vi "Teleop.vi"(10 "Match Info":T1={"Autonomous Elapsed Seconds"=0.0, "TeleOp Elapsed Seconds"=0.0, "Disabled Elapsed Seconds"=0.0, "Visited Autonomous"=FALSE, "Visited TeleOp"=FALSE, "Visited Disabled"=FALSE, "Autonomous Settings"={"Autonomous Style"=enum."Independent", "VI Refnum"=refnum}}, 11 "Call Context":T2) -> ()   [LabVIEW 2017]
doc: "This VI is called for each TeleOp packet received from the DS where the robot is not disabled. It is often used to read from the joysticks and update I/O or to update setpoints for timed control loops. It should complete and return within 20 milliseconds or it may miss DS packets."
uses:
  <vilib>/Rock Robotics/WPI/DriverStation/WPI_DriverStationDerivedRobotMode.ctl
  <vilib>/Rock Robotics/WPI/DriverStation/WPI_DriverStationMatch Info.ctl
  <vilib>/Rock Robotics/WPI/Solenoid/WPI_SolenoidValue.ctl
  <vilib>/Rock Robotics/WPI/Utilities/WPI_GetSetVariantRefNum.vi
  <vilib>/Rock Robotics/Network Tables/NT Write Boolean Array.vi
  <vilib>/Rock Robotics/Network Tables/NT Write Numeric Array.vi
  <vilib>/Rock Robotics/Network Tables/NT Read Boolean.vi
  <vilib>/Rock Robotics/Network Tables/NT Read Number.vi
  Robot Global Data.vi
  <vilib>/Rock Robotics/WPI/ThirdParty/Phoenix-LabVIEW/Motor Controller/Get/CTRE_Phoenix_MotorController_GetQuadratureData.vi
  <vilib>/Rock Robotics/WPI/Solenoid/WPI_SolenoidSetEnum.vi
  <vilib>/Rock Robotics/WPI/RobotDrive/WPI_RobotDriveArcadeDrive_Standard(NoSaturation).vi
panel:
  out "Quadrature Velocity":i32
  out "height":dbl
  out "Quadrature Position":i32
  out "Sample Slider 0":dbl(slide) scale=0.0..5.0
  out "Sample Boolean 1":bool
  out "Sample Boolean 0":bool
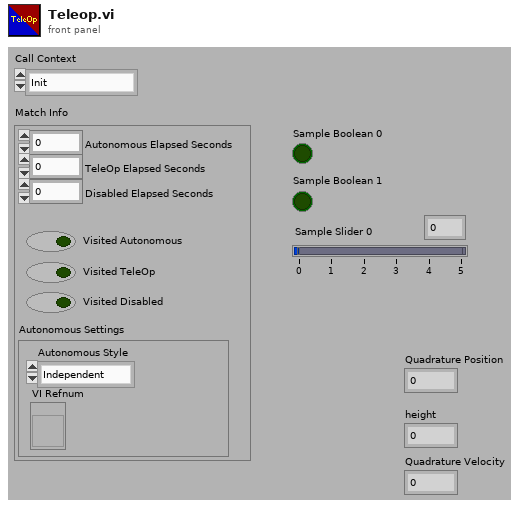
[diagram p1: front panel]
types:
  T1 = typedef "WPI_DriverStationMatch Info.ctl" = cluster{"Autonomous Elapsed Seconds":dbl, "TeleOp Elapsed Seconds":dbl, "Disabled Elapsed Seconds":dbl, "Visited Autonomous":bool, "Visited TeleOp":bool, "Visited Disabled":bool, "Autonomous Settings":cluster{"Autonomous Style":enum16{"Iterative", "Independent"}, "VI Refnum":refnum<vi>}}
  T2 = typedef "WPI_DriverStationDerivedRobotMode.ctl" = enum16{"Init", "Execute", "Stop"}
  T3 = typedef "WPI_SolenoidValue.ctl" = enum16{"Off", "On", "Forward", "Reverse"}
  T4 = typedef "WPI_JoystickDevRef.ctl" = cluster{"Device":T5}
  T5 = typedef "WPI_JoystickDeviceEnum.ctl" = enum16{"USB 0", "USB 1", "USB 2", "USB 3", "USB 4", "USB 5"}
  T6 = typedef "WPI_RobotDriveDevRef.ctl" = cluster{"DevStatus":errorcluster, "Motors[]":T7[], "Square Inputs":bool, "Max Output":dbl}
  T7 = typedef "WPI_MotorControlDeviceRef.ctl" = cluster{"DeviceStatus":errorcluster, "Type":T8, "PWM":cluster{"PWM Channel":T9, "DeadBand":T10}, "CAN":cluster{"Device Number":u8, "SetOutput VI Ref":variant, "GetOutput VI Ref":variant, "Enable VI Ref":variant, "Disable VI Ref":variant, "Data":variant}, "Invert":bool, "DIO PWM":cluster{"PWM \"Enable\" Channel":T9, "DIOChannel":T11, "PWM Rate":dbl}}
  T8 = typedef "WPI_MotorControlType.ctl" = enum16{"PWM", "CAN", "DIO PWM"}
  T9 = typedef "FPGA_DIOPWMChannel.ctl" = enum8{"PWM 0", "PWM 1", "PWM 2", "PWM 3", "PWM 4", "PWM 5", "PWM 6", "PWM 7", "PWM 8", "PWM 9", "PWM MXP 0", "PWM MXP 1", "PWM MXP 2", "PWM MXP 3", "PWM MXP 4", "PWM MXP 5", "PWM MXP 6", "PWM MXP 7", "PWM MXP 8", "PWM MXP 9", "Invalid"}
  T10 = typedef "WPI_PWMDeadband.ctl" = cluster{"Name":string, "maxPositivePwm":i32, "minPositivePwm":i32, "centerPwm":i32, "maxNegativePwm":i32, "minNegativePwm":i32, "angularRange":u16}
  T11 = typedef "FPGA_DIOChannel.ctl" = enum8{"DIO 0", "DIO 1", "DIO 2", "DIO 3", "DIO 4", "DIO 5", "DIO 6", "DIO 7", "DIO 8", "DIO 9", "DIO MXP 0", "DIO MXP 1", "DIO MXP 2", "DIO MXP 3", "DIO MXP 4", "DIO MXP 5", "DIO MXP 6", "DIO MXP 7", "DIO MXP 8", "DIO MXP 9", "DIO MXP 10", "DIO MXP 11", "DIO MXP 12", "DIO MXP 13", "DIO MXP 14", "DIO MXP 15", "SPI Port CS1", "SPI Port CS2", "SPI Port CS3", "SPI Port MISO", "SPI Port MOSI", "Invalid"}
  T12 = cluster{"Yaw":dbl, "Roll":dbl, "Pitch":dbl, "Heading":dbl, "Fused Heading":dbl}
  T13 = typedef "WPI_SolenoidDevRef.ctl" = cluster{"DevStatus":errorcluster, "Pneumatics Control Module":u8, "Forward Solenoid Channel":T14, "Reverse Solenoid Channel":T14}
  T14 = typedef "WPI_SolenoidChannel.ctl" = enum8{"Solenoid 0", "Solenoid 1", "Solenoid 2", "Solenoid 3", "Solenoid 4", "Solenoid 5", "Solenoid 6", "Solenoid 7", "Invalid"}
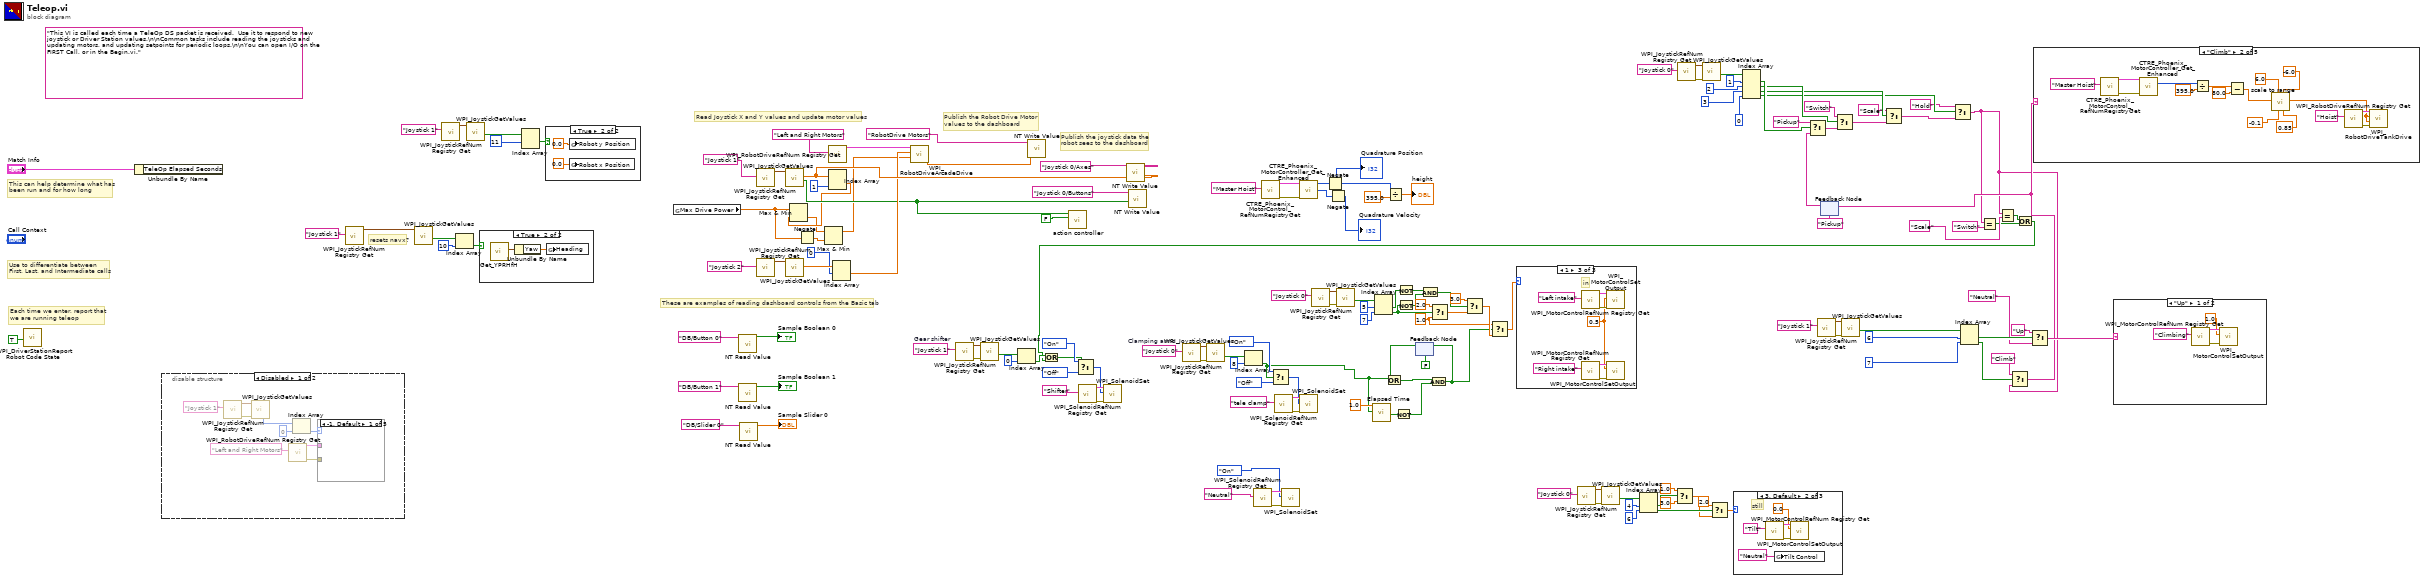
[diagram p0: block diagram]
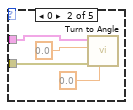
[diagram p2: hidden frame]
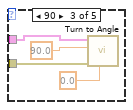
[diagram p3: hidden frame]
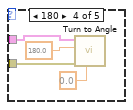
[diagram p4: hidden frame]
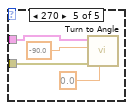
[diagram p5: hidden frame]
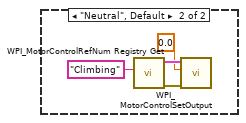
[diagram p7: hidden frame]
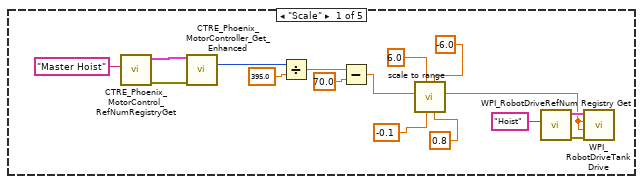
[diagram p8: hidden frame]
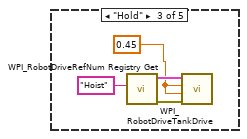
[diagram p9: hidden frame]
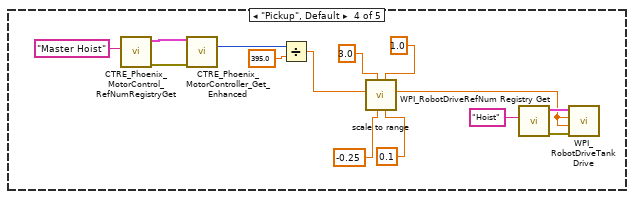
[diagram p10: hidden frame]
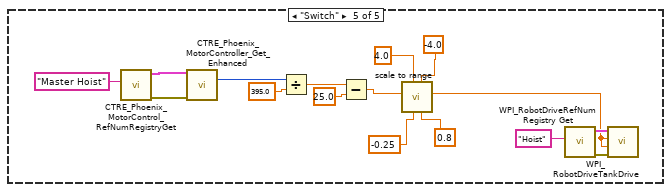
[diagram p11: hidden frame]
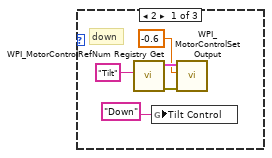
[diagram p12: hidden frame]
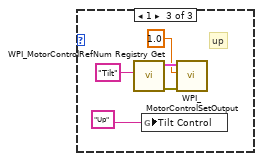
[diagram p13: hidden frame]
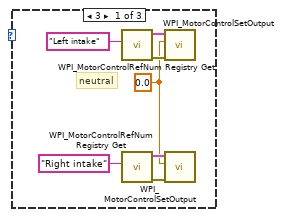
[diagram p14: hidden frame]
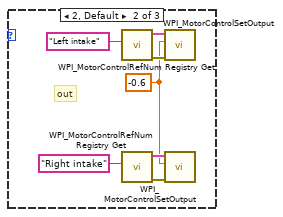
[diagram p15: hidden frame]
diagram:
  w74 = "Joystick 0"  # Clamping arms
  w65 = 1.0 ("f")
  w122 = "Joystick 1"  # Gear shifter
  (unwired) "This VI is called each time a TeleOp DS packet is received.  Use it to respond to new joystick or Driver Station values.\n\nCommon tasks include reading the joysticks and updating motors, and updating setpoints for periodic loops.\n\nYou can open I/O on the FIRST Call, or in the Begin.vi."
  # "resets navx?"
  # "These are examples of reading dashboard controls from the Basic tab"
  # "Publish the Robot Drive Motor\nvalues to the dashboard"
  # "Publish the joystick data the\nrobot sees to the dashboard"
  # "Each time we enter, report that\nwe are running teleop"
  # "Use to differentiate between\nFirst, Last, and Intermediate calls"
  # "This can help determine what has\nbeen run and for how long"
  # "Read Joystick X and Y values and update motor values"
  n1 = call <vilib>:"WPI_DriverStationReport Robot Code State.vi"("TeleOp"=TRUE ("Autonomous")) -> ()  [unwired: 10 in, 1 out]
  n2 = Unbundle By Name("Match Info") -> ()  [unwired: 1 out]
  n3 = disable-structure shown="Disabled" {
    frame Disabled {
      n4 = call <vilib>:"WPI_JoystickRefNum Registry Get.vi"("refnum name"="Joystick 1") -> ("error out"=w156:errorcluster, "JoystickDevRef"=w163:T4)  [unwired: 1 in, 8 out]
      n5 = call <vilib>:"WPI_JoystickGetValues.vi"("error in (no error)"=w156, "JoystickDevRef"=w163) -> ("POVs"=w157:i16[])  [unwired: 5 in, 4 out]
      n6 = call <vilib>:"WPI_RobotDriveRefNum Registry Get.vi"("refnum name"="Left and Right Motors") -> ("error out"=w160:errorcluster, "RobotDriveDevRef"=w159:T6)  [unwired: 1 in, 8 out]
      n7 = Index Array(array=w157, index=0) -> (element=w158:i16)
      n8 = case shown="-1, Default" w158 {
        tunnel: w160 -> [_ w166 w169 w175 w178]
        tunnel: w159 -> [_ w165 w170 w174 w177]
        frame -1, Default {
        }
        frame 0 {
          n9 = call "Turn to Angle.vi"("in power"=0.0, "error in (no error)"=w166, "Angle"=0.0, "RobotDriveDevRef"=w165) -> ()  [unwired: 5 in, 3 out]
        }
        frame 90 {
          n10 = call "Turn to Angle.vi"("in power"=0.0, "error in (no error)"=w169, "Angle"=90.0, "RobotDriveDevRef"=w170) -> ()  [unwired: 5 in, 3 out]
        }
        frame 180 {
          n11 = call "Turn to Angle.vi"("in power"=0.0, "error in (no error)"=w175, "Angle"=180.0, "RobotDriveDevRef"=w174) -> ()  [unwired: 5 in, 3 out]
        }
        frame 270 {
          n12 = call "Turn to Angle.vi"("in power"=0.0, "error in (no error)"=w178, "Angle"=-90.0, "RobotDriveDevRef"=w177) -> ()  [unwired: 5 in, 3 out]
        }
      }
    }
    frame Enabled {
    }
  }
  n13 = call <vilib>:"WPI_JoystickRefNum Registry Get.vi"("refnum name"="Joystick 1") -> ("JoystickDevRef"=w132:T4)  [unwired: 1 in, 9 out]
  n14 = call <vilib>:"WPI_JoystickGetValues.vi"("JoystickDevRef"=w132) -> ("Buttons"=w130:bool[])  [unwired: 6 in, 4 out]
  n15 = call <vilib>:"WPI_JoystickRefNum Registry Get.vi"("refnum name"="Joystick 1") -> ("JoystickDevRef"=w126:T4)  [unwired: 1 in, 9 out]
  n16 = Index Array(array=w130, index=10) -> (element=w129:bool)
  n17 = call <vilib>:"WPI_JoystickGetValues.vi"("JoystickDevRef"=w126) -> ("Buttons"=w124:bool[])  [unwired: 6 in, 4 out]
  n18 = case shown="True" w129 {
    frame False {
    }
    frame True {
      n19 = call <vilib>:"Get_YPRHfH.vi"() -> ("YRPHfH"=w182:T12)  [unwired: 11 in]
      n20 = Unbundle By Name(w182) -> ("Yaw"=w181:dbl)
      n21 = global write "Robot Global Data.vi" "Heading"(w181) -> ()
    }
  }
  n22 = Index Array(array=w124, index #1=11 ("index")) -> (element #1=w123:bool)  [unwired: 1 in, 1 out]
  n23 = case shown="True" w123 {
    frame False {
    }
    frame True {
      n24 = global write "Robot Global Data.vi" "Robot y Position"(0.0 ("Robot y Position")) -> ()
      n25 = global write "Robot Global Data.vi" "Robot x Position"(0.0 ("Robot x Position")) -> ()
    }
  }
  n26 = global read "Robot Global Data.vi" "Max Drive Power"() -> (w29:dbl)
  n27 = call-poly <vilib>:"NT Read Value.vi"("Name"="DB/Button 0" ("refnum name")) -> ("Boolean"=→"Sample Boolean 0":bool)  [unwired: 9 in, 1 out]
  n28 = call-poly <vilib>:"NT Read Value.vi"("Name"="DB/Button 1" ("refnum name")) -> ("Boolean"=→"Sample Boolean 1":bool)  [unwired: 9 in, 1 out]
  n29 = call-poly <vilib>:"NT Read Value.vi"("Name"="DB/Slider 0" ("refnum name")) -> ("Numeric"=→"Sample Slider 0":dbl)  [unwired: 9 in, 1 out]
  n30 = call <vilib>:"WPI_JoystickRefNum Registry Get.vi"("refnum name"="Joystick 1") -> ("JoystickDevRef"=w151:T4)  [unwired: 1 in, 9 out]
  n31 = call <vilib>:"WPI_JoystickRefNum Registry Get.vi"("refnum name"="Joystick 2") -> ("JoystickDevRef"=w136:T4)  [unwired: 1 in, 9 out]
  n32 = call <vilib>:"WPI_JoystickGetValues.vi"("JoystickDevRef"=w151) -> ("Buttons"=w78:bool[], "Axes"=w147:dbl[])  [unwired: 6 in, 3 out]
  n33 = call <vilib>:"WPI_JoystickGetValues.vi"("JoystickDevRef"=w136) -> ("Axes"=w135:dbl[])  [unwired: 6 in, 4 out]
  n34 = Negate(x=w29) -> (-x=w30:dbl)
  n35 = call <vilib>:"WPI_RobotDriveRefNum Registry Get.vi"("refnum name"="Left and Right Motors") -> ("RobotDriveDevRef"=w153:T6)  [unwired: 1 in, 9 out]
  n36 = Index Array(array=w147, index #1=1 ("index")) -> (element #1=w28:dbl)  [unwired: 1 in, 1 out]
  n37 = Max & Min(x=w29, y=w28) -> (min(x,y)=w27:dbl)  [unwired: 1 out]
  n38 = Max & Min(x=w27, y=w30) -> (max(x,y)=w26:dbl)  [unwired: 1 out]
  n39 = Index Array(array=w135, index #1=0 ("index")) -> (element #1=w112:dbl)  [unwired: 1 in, 1 out]
  n40 = call-poly <vilib>:"WPI_RobotDriveArcadeDrive.vi"("Y axis value"=w26, "X axis value"=w112, "RobotDriveDevRef"=w153) -> ("Motor Values"=w141:dbl[])  [unwired: 6 in, 2 out]
  n41 = call <vilib>:"WPI_JoystickRefNum Registry Get.vi"("refnum name"=w122) -> ("error out"=w81:errorcluster, "JoystickDevRef"=w121:T4)  [unwired: 1 in, 8 out]
  n42 = call <vilib>:"WPI_JoystickGetValues.vi"("error in (no error)"=w81, "JoystickDevRef"=w121) -> ("Buttons"=w119:bool[])  [unwired: 5 in, 4 out]
  n43 = Index Array(array=w119, index=0) -> (element=w15:bool)
  n44 = call-poly <vilib>:"NT Write Value.vi"("Numeric Array"=w141, "Name"="RobotDrive Motors") -> ()  [unwired: 9 in, 1 out]
  n45 = call "action controller.vi"("Box Sensor"=FALSE, "Buttons"=w78) -> ()  [unwired: 10 in]
  n46 = call <vilib>:"WPI_SolenoidRefNum Registry Get.vi"("refnum name"="Shifter") -> ("error out"=w118:errorcluster, "SolenoidDevRef"=w117:T13)  [unwired: 9 in]
  n47 = call-poly <vilib>:"NT Write Value.vi"("Numeric Array"=w147, "Name"="Joystick 0/Axes") -> ()  [unwired: 9 in, 1 out]
  n48 = call-poly <vilib>:"NT Write Value.vi"("Boolean Array"=w78, "Name"="Joystick 0/Buttons") -> ()  [unwired: 9 in, 1 out]
  n49 = call <vilib>:"WPI_JoystickRefNum Registry Get.vi"("refnum name"=w74) -> ("error out"=w72:errorcluster, "JoystickDevRef"=w73:T4)  [unwired: 1 in, 8 out]
  n50 = call <vilib>:"WPI_JoystickGetValues.vi"("error in (no error)"=w72, "JoystickDevRef"=w73) -> ("Buttons"=w71:bool[])  [unwired: 5 in, 4 out]
  n51 = Index Array(array=w71, index=8) -> (element=w1:bool)
  n52 = call <vilib>:"WPI_SolenoidRefNum Registry Get.vi"("refnum name"="Neutral") -> ("error out"=w6:errorcluster, "SolenoidDevRef"=w4:T13)  [unwired: 9 in]
  n53 = call <vilib>:"CTRE_Phoenix_MotorControl_RefNumRegistryGet.vi"("refnum name"="Master Hoist") -> ("error out"=w91:errorcluster, "PhoenixMotorControlDevRef"=w90:T7)  [unwired: 9 in]
  n54 = Select(t=WPI_SolenoidValue."On" ("Value"), s=w1, f=WPI_SolenoidValue."Off" ("Value")) -> (s? t:f=w67:T3)
  n55 = call <vilib>:"WPI_SolenoidRefNum Registry Get.vi"("refnum name"="tele clamp") -> ("error out"=w76:errorcluster, "SolenoidDevRef"=w77:T13)  [unwired: 9 in]
  n56 = call-poly <vilib>:"WPI_SolenoidSet.vi"("error in (no error)"=w6, "Value"=WPI_SolenoidValue."On", "SolenoidDevRef"=w4) -> ()  [unwired: 7 in, 2 out]
  n57 = call-poly <vilib>:"WPI_SolenoidSet.vi"("error in (no error)"=w76, "Value"=w67, "SolenoidDevRef"=w77) -> ()  [unwired: 7 in, 2 out]
  n58 = call-poly <vilib>:"CTRE_Phoenix_MotorController_Get_Enhanced.vi"("PhoenixMotorControlDevRef"=w90, "error in"=w91) -> ("Quadrature Position"=w87:i32, "Quadrature Velocity"=w62:i32)  [unwired: 10 in, 2 out]
  n59 = call <vilib>:"WPI_JoystickRefNum Registry Get.vi"("refnum name"="Joystick 0") -> ("error out"=w93:errorcluster, "JoystickDevRef"=w104:T4)  [unwired: 1 in, 8 out]
  n60 = Negate(x=w87) -> (-x=w40:i32)
  "Quadrature Position" <- w40
  n61 = Negate(x=w62) -> (-x=→"Quadrature Velocity":i32)
  n62 = call <vilib>:"WPI_JoystickGetValues.vi"("error in (no error)"=w93, "JoystickDevRef"=w104) -> ("Buttons"=w103:bool[])  [unwired: 5 in, 4 out]
  n63 = call "Elapsed Time"("Time Target (s)"=1.0, "Reset"=w1) -> ("Time has Elapsed"=w12:bool)  [unwired: 10 in, 7 out]
  n64 = Index Array(array=w103, index #1=5 ("index"), index #2=7 ("index")) -> (element #1=w101:bool, element #2=w95:bool)
  n65 = Divide(x=w40, y=395.0) -> (x/y=→"height":dbl)
  n66 = Not(x=w12) -> (.not. x?=w8:bool)
  n67 = Not(x=w101) -> (.not. x?=w100:bool)
  n68 = Not(x=w95) -> (.not. x?=w98:bool)
  n69 = feedback #1(FALSE) -> (w10:bool)
  n70 = Or(x=w1, y=w10) -> (x .or. y?=w9:bool)
  n71 = And(x=w100, y=w98) -> (x .and. y?=w99:bool)
  n72 = And(x=w9, y=w8) -> (x .and. y?=w7:bool)
  n73 = feedback-in #1(w7) -> ()
  n74 = Select(t=2.0, s=w95, f=w65) -> (s? t:f=w96:dbl)
  n75 = Select(t=3.0, s=w99, f=w96) -> (s? t:f=w66:dbl)
  n76 = Select(t=w65, s=w7, f=w66) -> (s? t:f=w64:dbl)
  n77 = case shown="1" w64 {
    frame 3 {
      w185 = 0.0
      # "neutral"
      n78 = call <vilib>:"WPI_MotorControlRefNum Registry Get.vi"("refnum name"="Left intake") -> ("error out"=w190:errorcluster, "MotorControlDevRef"=w189:T7)  [unwired: 9 in]
      n79 = call <vilib>:"WPI_MotorControlRefNum Registry Get.vi"("refnum name"="Right intake") -> ("error out"=w188:errorcluster, "MotorControlDevRef"=w187:T7)  [unwired: 9 in]
      n80 = call <vilib>:"WPI_MotorControlSetOutput.vi"("error in (no error)"=w190, "Output"=w185, "MotorControlDevRef"=w189) -> ()  [unwired: 6 in, 3 out]
      n81 = call <vilib>:"WPI_MotorControlSetOutput.vi"("error in (no error)"=w188, "Output"=w185, "MotorControlDevRef"=w187) -> ()  [unwired: 6 in, 3 out]
    }
    frame 2, Default {
      w192 = -0.6
      # "out"
      n82 = call <vilib>:"WPI_MotorControlRefNum Registry Get.vi"("refnum name"="Left intake") -> ("error out"=w197:errorcluster, "MotorControlDevRef"=w196:T7)  [unwired: 9 in]
      n83 = call <vilib>:"WPI_MotorControlRefNum Registry Get.vi"("refnum name"="Right intake") -> ("error out"=w195:errorcluster, "MotorControlDevRef"=w194:T7)  [unwired: 9 in]
      n84 = call <vilib>:"WPI_MotorControlSetOutput.vi"("error in (no error)"=w197, "Output"=w192, "MotorControlDevRef"=w196) -> ()  [unwired: 6 in, 3 out]
      n85 = call <vilib>:"WPI_MotorControlSetOutput.vi"("error in (no error)"=w195, "Output"=w192, "MotorControlDevRef"=w194) -> ()  [unwired: 6 in, 3 out]
    }
    frame 1 {
      w199 = 0.5 ("Output")
      # "in"
      n86 = call <vilib>:"WPI_MotorControlRefNum Registry Get.vi"("refnum name"="Left intake") -> ("error out"=w204:errorcluster, "MotorControlDevRef"=w203:T7)  [unwired: 9 in]
      n87 = call <vilib>:"WPI_MotorControlRefNum Registry Get.vi"("refnum name"="Right intake") -> ("error out"=w202:errorcluster, "MotorControlDevRef"=w201:T7)  [unwired: 9 in]
      n88 = call <vilib>:"WPI_MotorControlSetOutput.vi"("error in (no error)"=w204, "Output"=w199, "MotorControlDevRef"=w203) -> ()  [unwired: 6 in, 3 out]
      n89 = call <vilib>:"WPI_MotorControlSetOutput.vi"("error in (no error)"=w202, "Output"=w199, "MotorControlDevRef"=w201) -> ()  [unwired: 6 in, 3 out]
    }
  }
  n90 = call <vilib>:"WPI_JoystickRefNum Registry Get.vi"("refnum name"="Joystick 0") -> ("error out"=w106:errorcluster, "JoystickDevRef"=w110:T4)  [unwired: 1 in, 8 out]
  n91 = call <vilib>:"WPI_JoystickGetValues.vi"("error in (no error)"=w106, "JoystickDevRef"=w110) -> ("Buttons"=w109:bool[])  [unwired: 5 in, 4 out]
  n92 = Index Array(array=w109, index #1=4 ("index"), index #2=6 ("index")) -> (element #1=w86:bool, element #2=w85:bool)
  n93 = Select(t=1.0, s=w86, f=3.0) -> (s? t:f=w80:dbl)
  n94 = call <vilib>:"WPI_JoystickRefNum Registry Get.vi"("refnum name"="Joystick 0") -> ("error out"=w61:errorcluster, "JoystickDevRef"=w60:T4)  [unwired: 9 in]
  n95 = call <vilib>:"WPI_JoystickGetValues.vi"("error in (no error)"=w61, "JoystickDevRef"=w60) -> ("Buttons"=w57:bool[])  [unwired: 5 in, 4 out]
  n96 = Select(t=2.0 ("f"), s=w85, f=w80) -> (s? t:f=w82:dbl)
  n97 = case shown="3, Default" w82 {
    frame 2 {
      # "down"
      n98 = call <vilib>:"WPI_MotorControlRefNum Registry Get.vi"("refnum name"="Tilt") -> ("error out"=w209:errorcluster, "MotorControlDevRef"=w208:T7)  [unwired: 9 in]
      n99 = global write "Robot Global Data.vi" "Tilt Control"("Down") -> ()
      n100 = call <vilib>:"WPI_MotorControlSetOutput.vi"("error in (no error)"=w209, "Output"=-0.6, "MotorControlDevRef"=w208) -> ()  [unwired: 6 in, 3 out]
    }
    frame 3, Default {
      # "still"
      n101 = call <vilib>:"WPI_MotorControlRefNum Registry Get.vi"("refnum name"="Tilt") -> ("error out"=w214:errorcluster, "MotorControlDevRef"=w213:T7)  [unwired: 9 in]
      n102 = global write "Robot Global Data.vi" "Tilt Control"("Neutral") -> ()
      n103 = call <vilib>:"WPI_MotorControlSetOutput.vi"("error in (no error)"=w214, "Output"=0.0, "MotorControlDevRef"=w213) -> ()  [unwired: 6 in, 3 out]
    }
    frame 1 {
      # "up"
      n104 = call <vilib>:"WPI_MotorControlRefNum Registry Get.vi"("refnum name"="Tilt") -> ("error out"=w219:errorcluster, "MotorControlDevRef"=w218:T7)  [unwired: 9 in]
      n105 = global write "Robot Global Data.vi" "Tilt Control"("Up") -> ()
      n106 = call <vilib>:"WPI_MotorControlSetOutput.vi"("error in (no error)"=w219, "Output"=1.0, "MotorControlDevRef"=w218) -> ()  [unwired: 6 in, 3 out]
    }
  }
  n107 = Index Array(array=w57, index #1=1 ("index"), index #2=2 ("index"), index #3=3 ("index"), index #4=0 ("index")) -> (element #1=w54:bool, element #2=w52:bool, element #3=w51:bool, element #4=w22:bool)
  n108 = call <vilib>:"WPI_JoystickRefNum Registry Get.vi"("refnum name"="Joystick 1") -> ("error out"=w34:errorcluster, "JoystickDevRef"=w37:T4)  [unwired: 1 in, 8 out]
  n109 = feedback #2("Pickup") -> (w46:string)
  n110 = Select(t="Pickup", s=w54, f=w46) -> (s? t:f=w48:string)
  n111 = Select(t="Switch", s=w52, f=w48) -> (s? t:f=w47:string)
  n112 = call <vilib>:"WPI_JoystickGetValues.vi"("error in (no error)"=w34, "JoystickDevRef"=w37) -> ("Buttons"=w36:bool[])  [unwired: 5 in, 4 out]
  n113 = Select(t="Scale", s=w51, f=w47) -> (s? t:f=w21:string)
  n114 = Select(t="Hold", s=w22, f=w21) -> (s? t:f=w16:string)
  n115 = Index Array(array=w36, index #1=6 ("index"), index #2=7 ("index")) -> (element #1=w33:bool, element #2=w19:bool)
  n116 = Equal?(x=w16, y="Switch") -> (x = y?=w41:bool)
  n117 = Equal?(x=w16, y="Scale") -> (x = y?=w42:bool)
  n118 = Select(t="Climb", s=w19, f=w16) -> (s? t:f=w17:string)
  n119 = feedback-in #2(w17) -> ()
  n120 = Or(x=w42, y=w41) -> (x .or. y?=w14:bool)
  n121 = Or(x=w15, y=w14) -> (x .or. y?=w13:bool)
  n122 = Select(t=WPI_SolenoidValue."On" ("Value"), s=w13, f=WPI_SolenoidValue."Off" ("Value")) -> (s? t:f=w113:T3)
  n123 = call-poly <vilib>:"WPI_SolenoidSet.vi"("error in (no error)"=w118, "Value"=w113, "SolenoidDevRef"=w117) -> ()  [unwired: 7 in, 2 out]
  n124 = Select(t="Up", s=w33, f="Neutral") -> (s? t:f=w25:string)
  n125 = case shown="\"Climb\"" w17 {
    frame "Scale" {
      n126 = call <vilib>:"CTRE_Phoenix_MotorControl_RefNumRegistryGet.vi"("refnum name"="Master Hoist") -> ("error out"=w233:errorcluster, "PhoenixMotorControlDevRef"=w232:T7)  [unwired: 9 in]
      n127 = call-poly <vilib>:"CTRE_Phoenix_MotorController_Get_Enhanced.vi"("PhoenixMotorControlDevRef"=w232, "error in"=w233) -> ("Quadrature Position"=w222:i32)  [unwired: 10 in, 3 out]
      n128 = Divide(x=w222, y=395.0) -> (x/y=w229:dbl)
      n129 = Subtract(x=w229, y=70.0) -> (x-y=w227:dbl)
      n130 = call "scale to range.vi"("Max"=0.8, "High"=-6.0, "Min"=-0.1, "Low"=6.0, "In Signal"=w227) -> ("Output signal"=w221:dbl)  [unwired: 6 in]
      n131 = call <vilib>:"WPI_RobotDriveRefNum Registry Get.vi"("refnum name"="Hoist") -> ("error out"=w236:errorcluster, "RobotDriveDevRef"=w234:T6)  [unwired: 9 in]
      n132 = call <vilib>:"WPI_RobotDriveTankDrive.vi"("error in (no error)"=w236, "Right axis value"=w221, "Left axis value"=w221, "RobotDriveDevRef"=w234) -> ()  [unwired: 5 in, 3 out]
    }
    frame "Climb" {
      n133 = call <vilib>:"CTRE_Phoenix_MotorControl_RefNumRegistryGet.vi"("refnum name"="Master Hoist") -> ("error out"=w249:errorcluster, "PhoenixMotorControlDevRef"=w248:T7)  [unwired: 9 in]
      n134 = call-poly <vilib>:"CTRE_Phoenix_MotorController_Get_Enhanced.vi"("PhoenixMotorControlDevRef"=w248, "error in"=w249) -> ("Quadrature Position"=w238:i32)  [unwired: 10 in, 3 out]
      n135 = Divide(x=w238, y=395.0) -> (x/y=w245:dbl)
      n136 = Subtract(x=w245, y=80.0) -> (x-y=w243:dbl)
      n137 = call "scale to range.vi"("Max"=0.85, "High"=-6.0, "Min"=-0.1, "Low"=6.0, "In Signal"=w243) -> ("Output signal"=w237:dbl)  [unwired: 6 in]
      n138 = call <vilib>:"WPI_RobotDriveRefNum Registry Get.vi"("refnum name"="Hoist") -> ("error out"=w252:errorcluster, "RobotDriveDevRef"=w250:T6)  [unwired: 9 in]
      n139 = call <vilib>:"WPI_RobotDriveTankDrive.vi"("error in (no error)"=w252, "Right axis value"=w237, "Left axis value"=w237, "RobotDriveDevRef"=w250) -> ()  [unwired: 5 in, 3 out]
    }
    frame "Hold" {
      w253 = 0.45 ("Left axis value")
      n140 = call <vilib>:"WPI_RobotDriveRefNum Registry Get.vi"("refnum name"="Hoist") -> ("error out"=w256:errorcluster, "RobotDriveDevRef"=w254:T6)  [unwired: 9 in]
      n141 = call <vilib>:"WPI_RobotDriveTankDrive.vi"("error in (no error)"=w256, "Right axis value"=w253, "Left axis value"=w253, "RobotDriveDevRef"=w254) -> ()  [unwired: 5 in, 3 out]
    }
    frame "Pickup", Default {
      n142 = call <vilib>:"CTRE_Phoenix_MotorControl_RefNumRegistryGet.vi"("refnum name"="Master Hoist") -> ("error out"=w268:errorcluster, "PhoenixMotorControlDevRef"=w267:T7)  [unwired: 9 in]
      n143 = call-poly <vilib>:"CTRE_Phoenix_MotorController_Get_Enhanced.vi"("PhoenixMotorControlDevRef"=w267, "error in"=w268) -> ("Quadrature Position"=w257:i32)  [unwired: 10 in, 3 out]
      n144 = Divide(x=w257, y=395.0) -> (x/y=w259:dbl)
      n145 = call "scale to range.vi"("Max"=0.1, "High"=1.0, "Min"=-0.25, "Low"=3.0, "In Signal"=w259) -> ("Output signal"=w258:dbl)  [unwired: 6 in]
      n146 = call <vilib>:"WPI_RobotDriveRefNum Registry Get.vi"("refnum name"="Hoist") -> ("error out"=w270:errorcluster, "RobotDriveDevRef"=w264:T6)  [unwired: 9 in]
      n147 = call <vilib>:"WPI_RobotDriveTankDrive.vi"("error in (no error)"=w270, "Right axis value"=w258, "Left axis value"=w258, "RobotDriveDevRef"=w264) -> ()  [unwired: 5 in, 3 out]
    }
    frame "Switch" {
      n148 = call <vilib>:"CTRE_Phoenix_MotorControl_RefNumRegistryGet.vi"("refnum name"="Master Hoist") -> ("error out"=w284:errorcluster, "PhoenixMotorControlDevRef"=w283:T7)  [unwired: 9 in]
      n149 = call-poly <vilib>:"CTRE_Phoenix_MotorController_Get_Enhanced.vi"("PhoenixMotorControlDevRef"=w283, "error in"=w284) -> ("Quadrature Position"=w272:i32)  [unwired: 10 in, 3 out]
      n150 = Divide(x=w272, y=395.0) -> (x/y=w279:dbl)
      n151 = Subtract(x=w279, y=25.0) -> (x-y=w273:dbl)
      n152 = call "scale to range.vi"("Max"=0.8, "High"=-4.0, "Min"=-0.25, "Low"=4.0, "In Signal"=w273) -> ("Output signal"=w274:dbl)  [unwired: 6 in]
      n153 = call <vilib>:"WPI_RobotDriveRefNum Registry Get.vi"("refnum name"="Hoist") -> ("error out"=w286:errorcluster, "RobotDriveDevRef"=w280:T6)  [unwired: 9 in]
      n154 = call <vilib>:"WPI_RobotDriveTankDrive.vi"("error in (no error)"=w286, "Right axis value"=w274, "Left axis value"=w274, "RobotDriveDevRef"=w280) -> ()  [unwired: 5 in, 3 out]
    }
  }
  n155 = case shown="\"Up\"" w25 {
    frame "Up" {
      n156 = call <vilib>:"WPI_MotorControlRefNum Registry Get.vi"("refnum name"="Climbing") -> ("error out"=w290:errorcluster, "MotorControlDevRef"=w289:T7)  [unwired: 9 in]
      n157 = call <vilib>:"WPI_MotorControlSetOutput.vi"("error in (no error)"=w290, "Output"=1.0, "MotorControlDevRef"=w289) -> ()  [unwired: 6 in, 3 out]
    }
    frame "Neutral", Default {
      n158 = call <vilib>:"WPI_MotorControlRefNum Registry Get.vi"("refnum name"="Climbing") -> ("error out"=w294:errorcluster, "MotorControlDevRef"=w293:T7)  [unwired: 9 in]
      n159 = call <vilib>:"WPI_MotorControlSetOutput.vi"("error in (no error)"=w294, "Output"=0.0, "MotorControlDevRef"=w293) -> ()  [unwired: 6 in, 3 out]
    }
  }
